vi "Text2013.vi"   [LabVIEW 2013]
uses:
  <vilib>/Heliosphere Research LLC/Advanced Plotting Toolkit/api_annotations/TextProperties.ctl
  <vilib>/Heliosphere Research LLC/Advanced Plotting Toolkit/properties/Text.ctl
  <vilib>/Heliosphere Research LLC/Advanced Plotting Toolkit/typedefs/PlotColor.ctl
  <vilib>/Heliosphere Research LLC/Advanced Plotting Toolkit/properties/Text_FontSize.ctl
  <vilib>/Heliosphere Research LLC/Advanced Plotting Toolkit/properties/Text_FontStyle.ctl
  <vilib>/Heliosphere Research LLC/Advanced Plotting Toolkit/properties/Display.ctl
  ModeType.ctl
  <vilib>/Heliosphere Research LLC/Advanced Plotting Toolkit/Advanced Plotting Toolkit.lvlib
types:
  T1 = typedef "ModeType.ctl" = enum16{"Normal", "Expected Failure", "Skipped", "Broken"}
  T2 = typedef "Advanced Plotting Toolkit.lvlib/TextProperties.ctl" = cluster{"Text":T3, "Display":T7}
  T3 = typedef "Advanced Plotting Toolkit.lvlib/Text.ctl" = cluster{"Color":T4, "Background Color":T4, "Font Size (points)":T5, "Font Style":T6, "Rotation Angle":dbl}
  T4 = typedef "Advanced Plotting Toolkit.lvlib/PlotColor.ctl" = u32
  T5 = typedef "Advanced Plotting Toolkit.lvlib/Text_FontSize.ctl" = i32
  T6 = typedef "Advanced Plotting Toolkit.lvlib/Text_FontStyle.ctl" = enum16{"Automatic", "Normal", "Italic", "Bold"}
  T7 = typedef "Advanced Plotting Toolkit.lvlib/Display.ctl" = cluster{"Alpha":dbl, "Z Order":dbl}
  T8 = typedef "Advanced Plotting Toolkit.lvlib/PlotID.ctl" = i32
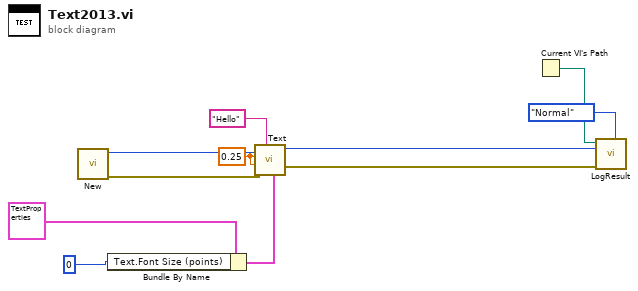
[diagram p0: block diagram]
diagram:
  w10 = 0.25 ("X Position")
  n1 = call <vilib>:"New.vi"() -> ("error out"=w7:errorcluster, "Plot ID"=w8:T8)  [unwired: 10 in]
  n2 = Bundle By Name(cluster=T2 {"Text"={"Color"=2147483647, "Background Color"=2147483647, "Font Size (points)"=0, "Font Style"=enum."Automatic", "Rotation Angle"=nan}, "Display"={"Alpha"=nan, "Z Order"=nan}} ("Text Properties"), "Text.Font Size (points)"=0) -> (w3:T2)
  n3 = call <vilib>:"Text.vi"("Properties"=w3, "Text"="Hello", "error in (no error)"=w7, "Y Position"=w10, "X Position"=w10, "Plot ID"=w8) -> ("error out"=w5:errorcluster, "Plot ID Out"=w6:T8)  [unwired: 4 in]
  n4 = Current VI's Path() -> (path=w11:path)
  n5 = call "LogResult.vi"("Mode"=ModeType."Normal", "Test Result"=w5, "Test Artifact"=w6, "VI Path"=w11) -> ()  [unwired: 8 in]
